vi "FRCts20_WebMethods_EspEngine.vi"(8 "error in (no error)":errorcluster, 9 "Cluster":variant, 10 "Return Type":T1="mobile", 11 "httpRequestID":u32) -> (0 "error out":errorcluster, 3 "httpRequestID out":u32)   [LabVIEW 2014]
doc: "Scripts the proper html for the provided <B>Cluster</B>. If the resource does not have a registered ESP page, XML will be output, assuming the client accepts XML data."
uses:
  Backend/source/VI Source/FRCts20_Backend_API/FRCts20_Backend_API_Team.ctl
  Backend/source/VI Source/FRCts20_Backend_API/FRCts20_Backend_API.lvlib
  Backend/source/VI Source/FRCts20_Backend_API/FRCts20_Backend_API_Request.ctl
  <vilib>/wsapi/NI_WebServices.lvlib
  <vilib>/regexp/Match Regular Expression.xnode
  FRCts20_WebMethods.lvlib
  Backend/source/VI Source/FRCts20_Backend_API/FRCts20_Backend_API_Status.ctl
  Backend/source/VI Source/FRCts20_Backend_API/FRCts20_Backend_API_SW.ctl
  <vilib>/wsapi/subVIs/Set String ESP Variable.vi
  Controls/FRCts20_WebMethods_Globals.vi
  Backend/source/VI Source/FRCts20_Backend_API/FRCts20_Backend_API_Note.ctl
  Controls/FRCts20_WebMethods_ctl_requestarray.ctl
  Controls/FRCts20_WebMethods_ctl_teamarray.ctl
  <vilib>/wsapi/subVIs/Set Integer ESP Variable.vi
  Backend/source/VI Source/FRCts20_Backend_API/FRCts20_Backend_API_Command_Competition.ctl
  Backend/source/VI Source/FRCts20_Backend_API/FRCts20_Backend_API_Competition.ctl
  Backend/source/VI Source/INI_Accessor/FRCts20_Backend_INI Controller.lvclass
  Backend/source/VI Source/FRCts20_Backend_API/FRCts20_Backend_API_Event.vi
  Controls/FRCts20_WebMethods_ctl_returntype.ctl
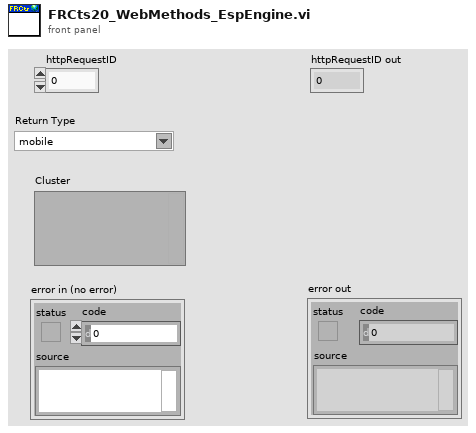
[diagram p1: front panel]
types:
  T1 = typedef "FRCts20_WebMethods.lvlib/FRCts20_WebMethods_ctl_returntype.ctl" = string
  T2 = typedef "FRCts20_Backend_API.lvlib/FRCts20_Backend_API_Team.ctl" = cluster{"Team Index":u32, "Team Number":u32, "Team Name":string, "Short Team Name":string, "Nick Name":string, "Robot Name":string, "City":string, "State":string, "Country":string, "Rookie Year":u32, "SWType":T3, "CAN":bool, "Vision":bool, "Kinect":bool, "Tags":string, "Avatar":string, "Request Array":cluster{"Request Index":u32, "Description":string, "Status":T4, "Open Date":timestamp, "Last Update":timestamp, "Close Date":timestamp}[], "Events Attending":cluster{"EventIndex":dbl, "EventName":string, "IsLive":bool}[], "APIReturn":string}
  T3 = typedef "FRCts20_Backend_API.lvlib/FRCts20_Backend_API_SW.ctl" = string
  T4 = typedef "FRCts20_Backend_API.lvlib/FRCts20_Backend_API_Status.ctl" = enum16{"Open", "In Work", "Closed"}
  T5 = typedef "FRCts20_Backend_API.lvlib/FRCts20_Backend_API_Note.ctl" = cluster{"Note Index":u32, "Request Index":u32, "Author":string, "Time Entered":timestamp, "Text":string, "Solution":bool, "APIReturn":string}
  T6 = typedef "FRCts20_WebMethods.lvlib/FRCts20_WebMethods_ctl_requestarray.ctl" = cluster{"Request Array":cluster{"Request Index":u32, "Description":string, "Status":T4}[]}
  T7 = typedef "FRCts20_WebMethods.lvlib/FRCts20_WebMethods_ctl_teamarray.ctl" = cluster{"Team":u32[]}
  T8 = typedef "FRCts20_Backend_API.lvlib/FRCts20_Backend_API_Request.ctl" = cluster{"Request Index":u32, "Description":string, "Status":T4, "Open Date":timestamp, "Last Update":timestamp, "Closed Date":timestamp, "Notes":cluster{"Note Index":u32, "Text":string, "Time Entered":timestamp, "Author":string, "Solution":bool}[], "Team Index":u32, "APIReturn":string}
  T9 = typedef "FRCts20_Backend_API.lvlib/FRCts20_Backend_API_Competition.ctl" = cluster{"Name":string, "Start Date":timestamp, "Duration":u8, "Divisions":string[], "APIReturn":string}
  T10 = typedef "FRCts20_Backend_API.lvlib/FRCts20_Backend_API_Command_Competition.ctl" = string
  T11 = typedef "FRCts20_Backend_API.lvlib/FRCts20_Backend_API_Event.ctl" = cluster{"Event Index":u32, "Name":string, "Start Time":timestamp, "End Time":timestamp, "Teams":cluster{"Team Index":u32, "Team Number":u32, "Requests":cluster{"Request Number":u32, "Description":string}[], "Has Open Issue":bool}[], "SWType":T3, "APIReturn":string}
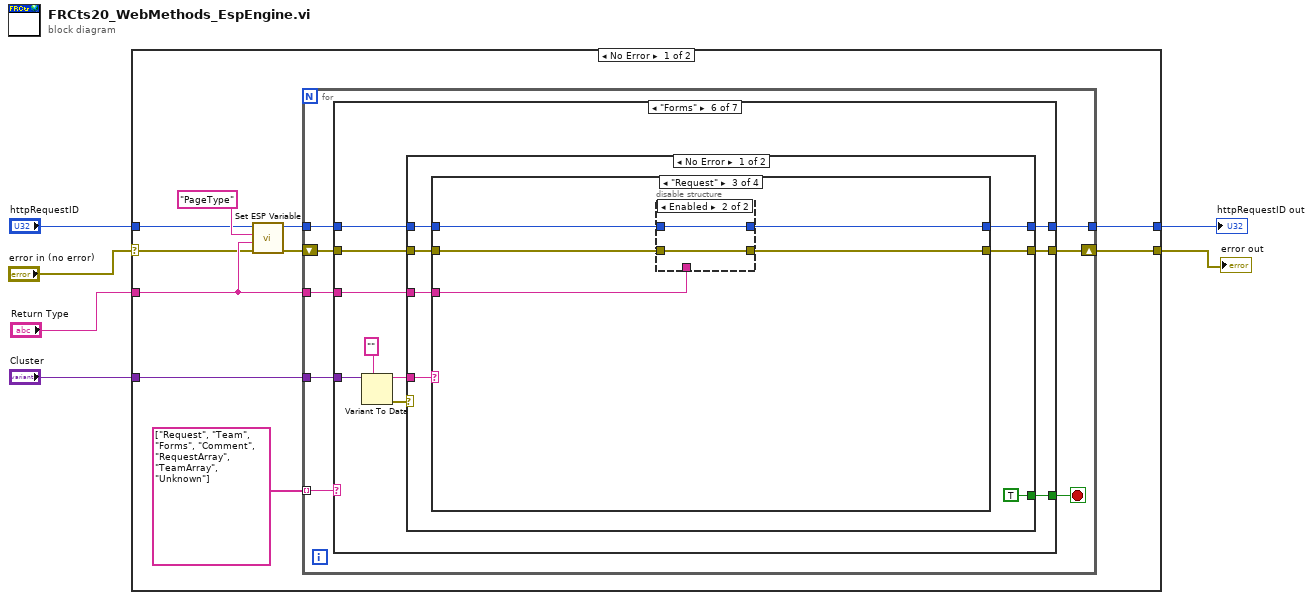
[diagram p0: block diagram]
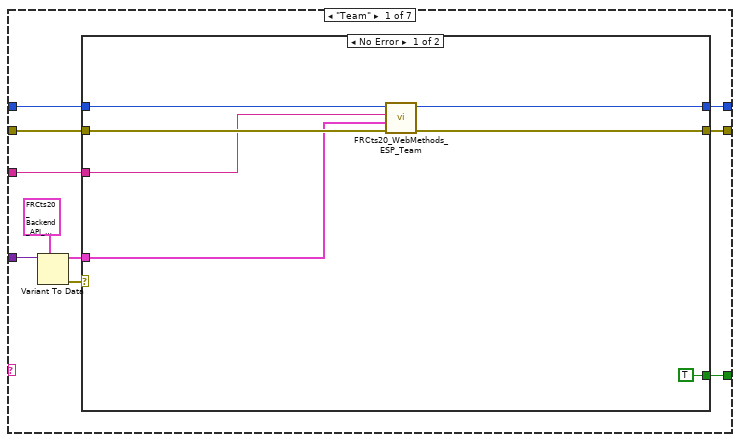
[diagram p2: hidden frame]
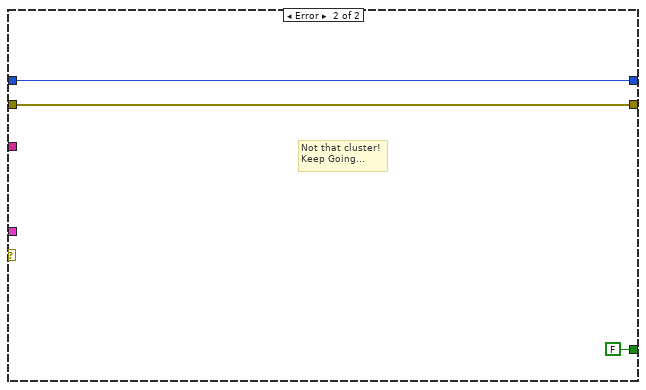
[diagram p3: hidden frame]
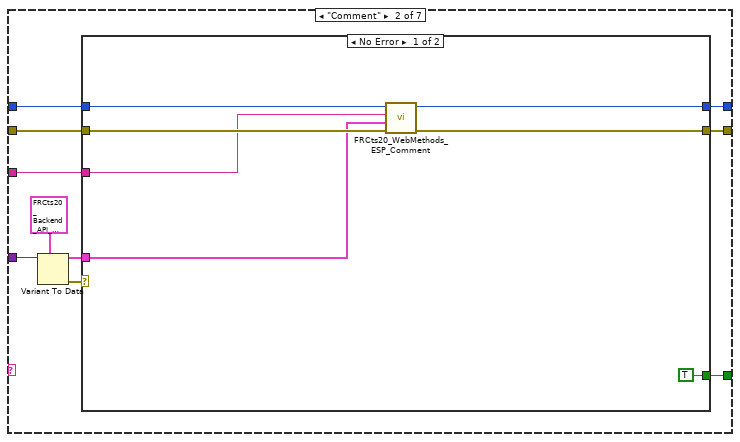
[diagram p4: hidden frame]
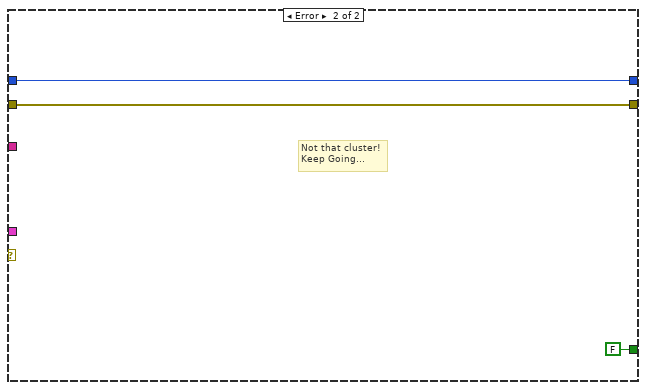
[diagram p5: hidden frame]
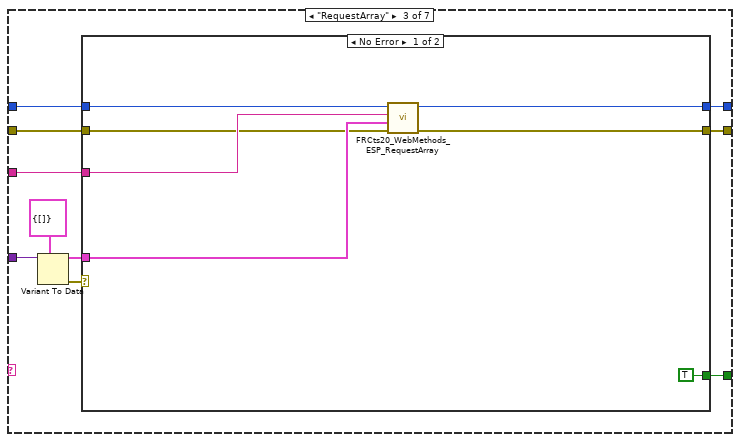
[diagram p6: hidden frame]
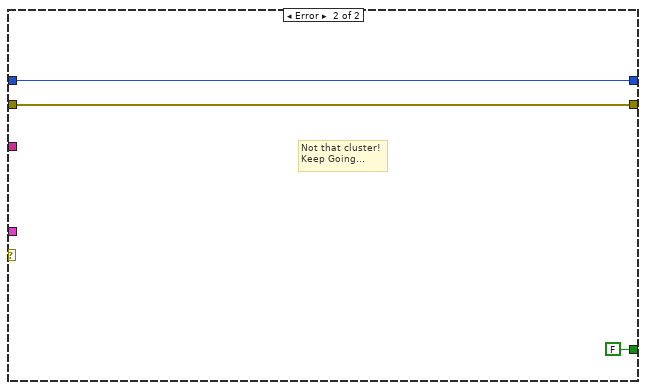
[diagram p7: hidden frame]
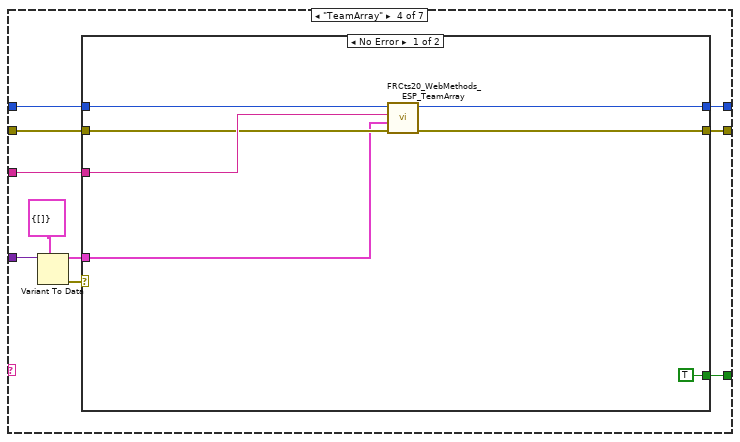
[diagram p8: hidden frame]
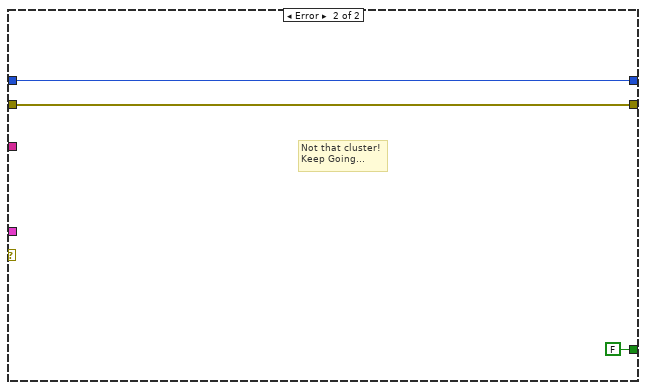
[diagram p9: hidden frame]
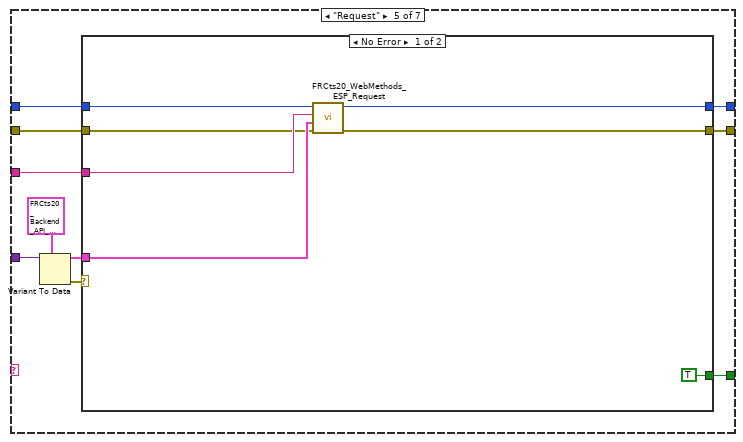
[diagram p10: hidden frame]
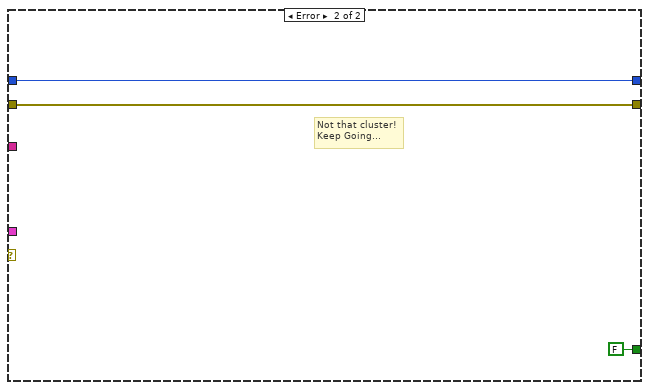
[diagram p11: hidden frame]
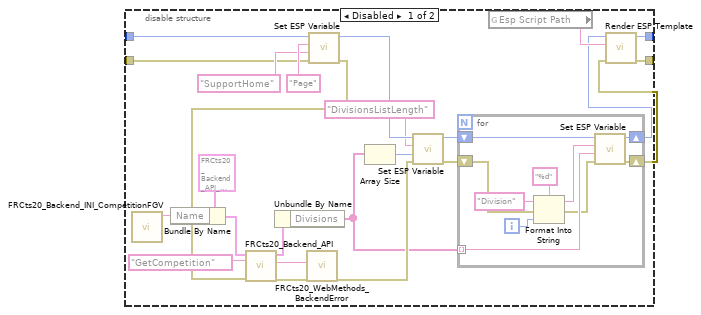
[diagram p14: hidden frame]
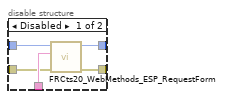
[diagram p15: hidden frame]
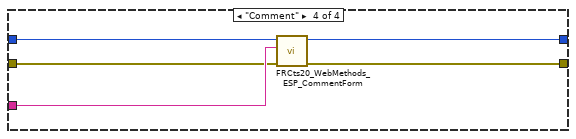
[diagram p16: hidden frame]
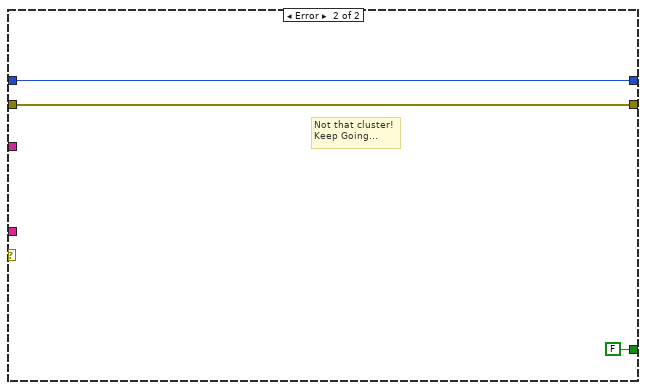
[diagram p17: hidden frame]
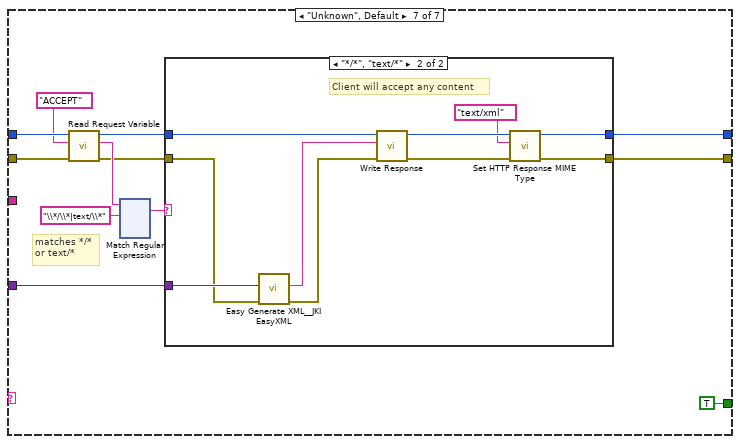
[diagram p18: hidden frame]
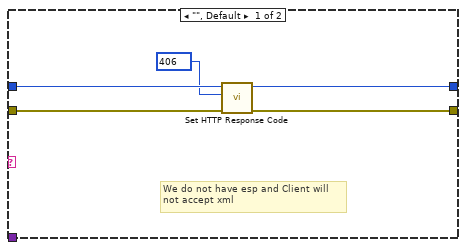
[diagram p19: hidden frame]
diagram:
  n1 = case shown="No Error" "error in (no error)" {
    selector: "error in (no error)" -> [w7 w342]
    tunnel: "Cluster" -> [w15 _]
    tunnel: "httpRequestID" -> [w8 w343]
    tunnel: [w14 w343] -> w4
    tunnel: [w13 w342] -> w2
    tunnel: "Return Type" -> [w10 _]
    frame No Error {
      n2 = call-poly <vilib>:"Set ESP Variable.vi"("error in (no error)"=w7, "value"=w10, "key"="PageType", "httpRequestID"=w8) -> ("error out"=w11:errorcluster, "httpRequestID out"=w12:u32)  [unwired: 6 in]
      n3 = for {
        tunnel: string[] ["Request", "Team", "Forms", "Comment", "RequestArray", "TeamArray", "Unknown"] -> [w24] mode=indexing
        tunnel: w15 -> [w23]
        tunnel: w12 -> [w21]
        tunnel: [w20] -> w14
        shift-right: [w19] -> w13
        shift-left: w11 -> [w18]
        tunnel: w10 -> [w17]
        stop <- w22 stop-if-true
        n4 = case shown="\"Forms\"" w24 {
          tunnel: w23 -> [w34 w54 w74 w94 w114 w134 w206]
          tunnel: [w30 w51 w71 w92 w111 w131 TRUE] -> w22
          tunnel: w21 -> [w29 w50 w70 w91 w109 w130 w214]
          tunnel: w18 -> [w28 w49 w69 w90 w108 w129 w212]
          tunnel: [w26 w47 w67 w88 w106 w127 w205] -> w19
          tunnel: [w27 w48 w68 w89 w107 w128 w204] -> w20
          tunnel: w17 -> [w25 w46 w66 w87 w105 w125 _]
          frame "Team" {
            n5 = Variant To Data(type=T2 {"Team Index"=0, "Team Number"=0, "Team Name"="", "Short Team Name"="", "Nick Name"="", "Robot Name"="", "City"="", "State"="", "Country"="", "Rookie Year"=0, "SWType"="", "CAN"=FALSE, "Vision"=FALSE, "Kinect"=FALSE, "Tags"="", "Avatar"="", "Request Array"=[], "Events Attending"=[], "APIReturn"=""} ("Team"), Variant=w34) -> (data=w31:T2, error out=w32:errorcluster)  [unwired: 1 in]
            n6 = case shown="No Error" w32 {
              tunnel: w31 -> [w36 _]
              tunnel: [TRUE FALSE] -> w30
              tunnel: w29 -> [w37 w43]
              tunnel: w28 -> [w38 w42]
              tunnel: [w39 w43] -> w27
              tunnel: [w40 w42] -> w26
              tunnel: w25 -> [w35 _]
              frame No Error {
                n7 = call "FRCts20_WebMethods_ESP_Team.vi"("error in (no error)"=w38, "Team"=w36, "Return Type"=w35, "httpRequestID"=w37) -> ("error out"=w40:errorcluster, "httpRequestID out"=w39:u32)  [unwired: 6 in]
              }
              frame Error {
                # "Not that cluster!\nKeep Going..."
              }
            }
          }
          frame "Comment" {
            n8 = Variant To Data(type=T5 {"Note Index"=0, "Request Index"=0, "Author"="", "Time Entered"=timestamp(0 s since 1904-01-01), "Text"="", "Solution"=FALSE, "APIReturn"=""} ("Note"), Variant=w54) -> (data=w52:T5, error out=w53:errorcluster)  [unwired: 1 in]
            n9 = case shown="No Error" w53 {
              tunnel: w52 -> [w55 _]
              tunnel: [TRUE FALSE] -> w51
              tunnel: w50 -> [w57 w63]
              tunnel: w49 -> [w58 w62]
              tunnel: [w59 w63] -> w48
              tunnel: [w60 w62] -> w47
              tunnel: w46 -> [w56 _]
              frame No Error {
                n10 = call "FRCts20_WebMethods_ESP_Comment.vi"("error in (no error)"=w58, "Note"=w55, "Return Type"=w56, "httpRequestID"=w57) -> ("error out"=w60:errorcluster, "httpRequestID out"=w59:u32)  [unwired: 6 in]
              }
              frame Error {
                # "Not that cluster!\nKeep Going..."
              }
            }
          }
          frame "RequestArray" {
            n11 = Variant To Data(type=T6 {"Request Array"=[]} ("Requests"), Variant=w74) -> (data=w72:T6, error out=w73:errorcluster)  [unwired: 1 in]
            n12 = case shown="No Error" w73 {
              tunnel: w72 -> [w76 _]
              tunnel: [TRUE FALSE] -> w71
              tunnel: w70 -> [w78 w83]
              tunnel: w69 -> [w75 w82]
              tunnel: [w79 w83] -> w68
              tunnel: [w80 w82] -> w67
              tunnel: w66 -> [w77 _]
              frame No Error {
                n13 = call "FRCts20_WebMethods_ESP_RequestArray.vi"("error in (no error)"=w75, "Requests"=w76, "Return Type"=w77, "httpRequestID"=w78) -> ("error out"=w80:errorcluster, "httpRequestID out"=w79:u32)  [unwired: 6 in]
              }
              frame Error {
                # "Not that cluster!\nKeep Going..."
              }
            }
          }
          frame "TeamArray" {
            n14 = Variant To Data(type=T7 {"Team"=[]} ("Teams"), Variant=w94) -> (data=w85:T7, error out=w93:errorcluster)  [unwired: 1 in]
            n15 = case shown="No Error" w93 {
              tunnel: [TRUE FALSE] -> w92
              tunnel: w91 -> [w98 w103]
              tunnel: w90 -> [w96 w102]
              tunnel: [w99 w103] -> w89
              tunnel: [w100 w102] -> w88
              tunnel: w87 -> [w97 _]
              tunnel: w85 -> [w95 _]
              frame No Error {
                n16 = call "FRCts20_WebMethods_ESP_TeamArray.vi"("error in (no error)"=w96, "Teams"=w95, "Return Type"=w97, "httpRequestID"=w98) -> ("error out"=w100:errorcluster, "httpRequestID out"=w99:u32)  [unwired: 6 in]
              }
              frame Error {
                # "Not that cluster!\nKeep Going..."
              }
            }
          }
          frame "Request" {
            n17 = Variant To Data(type=T8 {"Request Index"=0, "Description"="", "Status"=enum."Open", "Open Date"=timestamp(0 s since 1904-01-01), "Last Update"=timestamp(0 s since 1904-01-01), "Closed Date"=timestamp(0 s since 1904-01-01), "Notes"=[], "Team Index"=0, "APIReturn"=""} ("Request"), Variant=w114) -> (data=w112:T8, error out=w113:errorcluster)  [unwired: 1 in]
            n18 = case shown="No Error" w113 {
              tunnel: w112 -> [w117 _]
              tunnel: [TRUE FALSE] -> w111
              tunnel: w109 -> [w116 w122]
              tunnel: w108 -> [w115 w123]
              tunnel: [w120 w122] -> w107
              tunnel: [w119 w123] -> w106
              tunnel: w105 -> [w118 _]
              frame No Error {
                n19 = call "FRCts20_WebMethods_ESP_Request.vi"("error in (no error)"=w115, "Request"=w117, "Return Type"=w118, "httpRequestID"=w116) -> ("error out"=w119:errorcluster, "httpRequestID out"=w120:u32)  [unwired: 6 in]
              }
              frame Error {
                # "Not that cluster!\nKeep Going..."
              }
            }
          }
          frame "Forms" {
            n20 = Variant To Data(type="", Variant=w134) -> (data=w132:string, error out=w133:errorcluster)  [unwired: 1 in]
            n21 = case shown="No Error" w133 {
              tunnel: w132 -> [w140 _]
              tunnel: [TRUE FALSE] -> w131
              tunnel: w130 -> [w139 w201]
              tunnel: w129 -> [w138 w202]
              tunnel: [w136 w201] -> w128
              tunnel: [w137 w202] -> w127
              tunnel: w125 -> [w135 _]
              frame No Error {
                n22 = case shown="\"Request\"" w140 {
                  tunnel: w138 -> [w142 w146 w184 w196]
                  tunnel: w139 -> [w143 w147 w185 w197]
                  tunnel: [w142 w144 w186 w199] -> w137
                  tunnel: [w143 w145 w187 w200] -> w136
                  tunnel: w135 -> [_ _ w188 w198]
                  frame Default {
                  }
                  frame "Home" {
                    n23 = disable-structure shown="Enabled" {
                      disable-tunnel: w147 -> [w168 w183]
                      disable-tunnel: w146 -> [w167 w182]
                      disable-tunnel: [w166 w183] -> w145
                      disable-tunnel: [w165 w182] -> w144
                      frame Disabled {
                        n24 = call "FRCts20_Backend_INI_CompetitionFGV.vi"() -> ("Value out"=w163:string)  [unwired: 11 in]
                        n25 = Bundle By Name(cluster=T9 {"Name"="", "Start Date"=timestamp(0 s since 1904-01-01), "Duration"=0, "Divisions"=[], "APIReturn"=""} ("Competition In"), "Name"=w163) -> (w164:T9)
                        n26 = call-poly <vilib>:"Set ESP Variable.vi"("error in (no error)"=w167, "value"="SupportHome", "key"="Page", "httpRequestID"=w168) -> ("error out"=w152:errorcluster, "httpRequestID out"=w151:u32)  [unwired: 6 in]
                        n27 = call-poly "FRCts20_Backend_API.vi"("error in (no error)"=w152, "Command"=T10 "GetCompetition", "Event In"=w164) -> ("error out"=w159:errorcluster, "Status"=w160:string, "Event Out"=w153:T11)  [unwired: 6 in]
                        n28 = Unbundle By Name(w153) -> ("Divisions"=w155:string[])
                        n29 = call "FRCts20_WebMethods_BackendError.vi"("error in (no error)"=w159, "Status"=w160) -> ("error out"=w161:errorcluster)  [unwired: 8 in, 1 out]
                        n30 = Array Size(array=w155) -> (size(s)=w154:i32)
                        n31 = call-poly <vilib>:"Set ESP Variable.vi"("error in (no error)"=w161, "value"=w154, "key"="DivisionsListLength", "httpRequestID"=w151) -> ("error out"=w156:errorcluster, "httpRequestID out"=w157:u32)  [unwired: 6 in]
                        n32 = for {
                          tunnel: w155 -> [w176] mode=indexing
                          shift-right: [w181] -> w148
                          shift-left: w156 -> [w173]
                          shift-right: [w174] -> w149
                          shift-left: w157 -> [w180]
                          i -> [w178]
                          n33 = Format Into String(format string="%d", initial string="Division", error in=w173, w178) -> (resulting string=w177:string, error out=w172:errorcluster)
                          n34 = call-poly <vilib>:"Set ESP Variable.vi"("error in (no error)"=w172, "value"=w176, "key"=w177, "httpRequestID"=w180) -> ("error out"=w181:errorcluster, "httpRequestID out"=w174:u32)  [unwired: 6 in]
                        }
                        n35 = global read "FRCts20_WebMethods_Globals.vi" "Esp Script Path"() -> (w171:string)
                        n36 = call <vilib>:"Render ESP Template.vi"("error in (no error)"=w148, "espName"=w171, "httpRequestID"=w149) -> ("error out"=w165:errorcluster, "httpRequestID out"=w166:u32)  [unwired: 7 in]
                      }
                      frame Enabled {
                      }
                    }
                  }
                  frame "Request" {
                    n37 = disable-structure shown="Enabled" {
                      disable-tunnel: w188 -> [w193 _]
                      disable-tunnel: [w192 w195] -> w187
                      disable-tunnel: [w191 w194] -> w186
                      disable-tunnel: w185 -> [w190 w195]
                      disable-tunnel: w184 -> [w189 w194]
                      frame Disabled {
                        n38 = call "FRCts20_WebMethods_ESP_RequestForm.vi"("error in (no error)"=w189, "Return Type"=w193, "httpRequestID"=w190) -> ("error out"=w191:errorcluster, "httpRequestID out"=w192:u32)  [unwired: 7 in]
                      }
                      frame Enabled {
                      }
                    }
                  }
                  frame "Comment" {
                    n39 = call "FRCts20_WebMethods_ESP_CommentForm.vi"("error in (no error)"=w196, "Return Type"=w198, "httpRequestID"=w197) -> ("error out"=w199:errorcluster, "httpRequestID out"=w200:u32)  [unwired: 7 in]
                  }
                }
              }
              frame Error {
                # "Not that cluster!\nKeep Going..."
              }
            }
          }
          frame "Unknown", Default {
            # "matches */*\nor text/*"
            n40 = call <vilib>:"Read Request Variable.vi"("error in (no error)"=w212, "variable name"="ACCEPT", "httpRequestID"=w214) -> ("error out"=w208:errorcluster, "value"=w211:string, "httpRequestID out"=w207:u32)  [unwired: 6 in]
            n41 = xnode "Match Regular Expression"("input string"=w211, "regular expression"="\\*/\\*|text/\\*") -> ("whole match"=w209:string)  [unwired: 4 in, 4 out]
            n42 = case shown="\"*/*\", \"text/*\"" w209 {
              tunnel: w208 -> [w219 w227]
              tunnel: w207 -> [w220 w226]
              tunnel: w206 -> [_ w230]
              tunnel: [w218 w225] -> w205
              tunnel: [w217 w224] -> w204
              frame "", Default {
                w216 = 406 items=["100"=100, "101"=101, "200"=200, "201"=201, "202"=202, "203"=203, "204"=204, "205"=205, "206"=206, "300"=300, "301"=301, "302"=302, "303"=303, "304"=304, "305"=305, "306"=306, "307"=307, "400"=400, "401"=401, "402"=402, "403"=403, "404"=404, "405"=405, "406"=406, "407"=407, "408"=408, "409"=409, "410"=410, "411"=411, "412"=412, "413"=413, "414"=414, "415"=415, "416"=416, "417"=417, "500"=500, "501"=501, "502"=502, "503"=503, "504"=504, "505"=505] ("response code (200)")
                # "We do not have esp and Client will\nnot accept xml"
                n43 = call <vilib>:"Set HTTP Response Code.vi"("error in (no error)"=w219, "response code (200)"=w216, "httpRequestID"=w220) -> ("error out"=w218:errorcluster, "httpRequestID out"=w217:u32)  [unwired: 7 in]
              }
              frame "*/*", "text/*" {
                # "Client will accept any content"
                n44 = call <vilib>:"Easy Generate XML__JKI EasyXML.vi"("error in (no error)"=w227, "LabVIEW Data"=w230) -> ("error out"=w229:errorcluster, "XML String"=w228:string)  [unwired: 8 in]
                n45 = call <vilib>:"Write Response.vi"("error in (no error)"=w229, "response string"=w228, "httpRequestID"=w226) -> ("error out"=w223:errorcluster, "httpRequestID out"=w222:u32)  [unwired: 7 in]
                n46 = call <vilib>:"Set HTTP Response MIME Type.vi"("error in (no error)"=w223, "MIME type (text/html)"="text/xml", "httpRequestID"=w222) -> ("error out"=w225:errorcluster, "httpRequestID out"=w224:u32)  [unwired: 7 in]
              }
            }
          }
        }
      }
    }
    frame Error {
    }
  }
  "httpRequestID out" <- w4
  "error out" <- w2
